vi "1.2.1-SendReadRequest.vi"(10 "Command":u8[](array[numeric])=[0, 0, 0, 0, 0, 0, 0, 0, 0, 0, 0, 0]) -> (1 "Sending":bool, 2 "Serial Byte":u8)   [LabVIEW 2010]
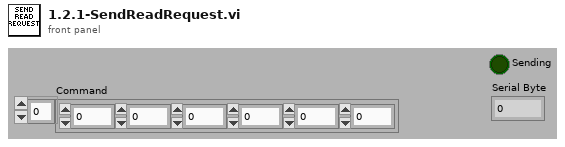
[diagram p1: front panel]
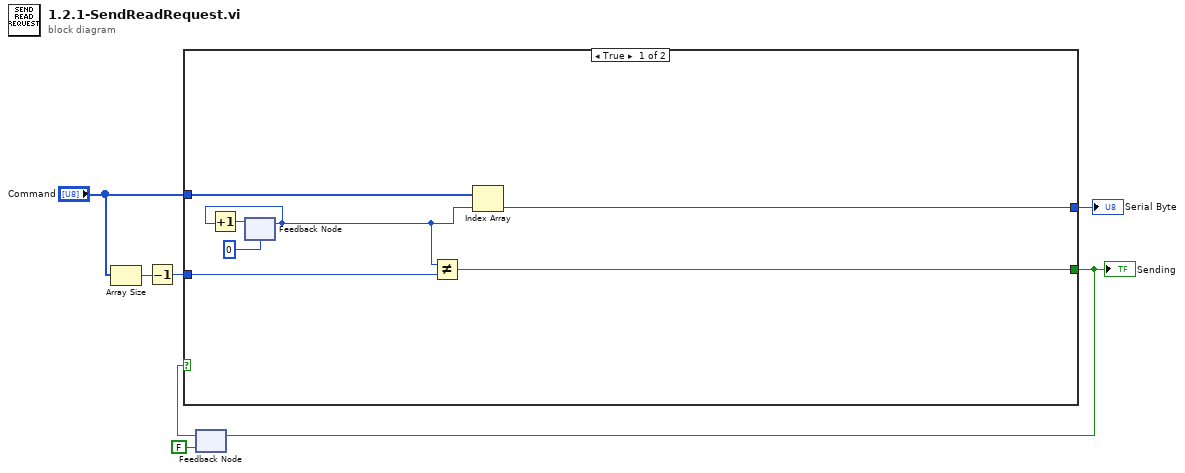
[diagram p0: block diagram]
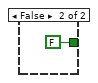
[diagram p2: hidden frame]
diagram:
  n1 = Array Size(array="Command") -> (size(s)=w5:i32)
  n2 = Decrement(x=w5) -> (x-1=w4:i32)
  n3 = feedback #1(FALSE) -> (w2:bool)
  n4 = case shown="True" w2 {
    tunnel: "Command" -> [w12 _]
    tunnel: [w11 _] -> w7
    tunnel: w4 -> [w10 _]
    tunnel: [w8 FALSE] -> w3
    frame True {
      n5 = feedback #2(0 ("Serial Byte")) -> (w9:i32)
      n6 = Increment(x=w9) -> (x+1=w13:i32)
      n7 = feedback-in #2(w13) -> ()
      n8 = Not Equal?(x=w9, y=w10) -> (x != y?=w8:bool)
      n9 = Index Array(array=w12, index=w9) -> (element=w11:u8)
    }
    frame False {
    }
  }
  "Serial Byte" <- w7
  "Sending" <- w3
  n10 = feedback-in #1(w3) -> ()
